vi "Stepper Motor Control.vi"() -> ()   [LabVIEW 2015]
uses:
  <vilib>/MakerHub/LINX/Public/Peripherals/Digital/Digital Write N Chans.vi
  <vilib>/MakerHub/LINX/Private/Local IO/LinxDigitalWrite.vi
  <vilib>/MakerHub/LINX/Public/Utilities/Check Channel.vi
  <vilib>/MakerHub/LINX/Public/Utilities/Open Serial.vi
  <vilib>/MakerHub/LINX/Private/Utilties/Generate Error.vi
  <vilib>/MakerHub/LINX/LMH-LINX.lvlib
panel:
  in  "States":bool[](array[boolean])
  in  "Serial Port":refnum<visa-resource-name>="COM12"
  in  "Stop":bool
  in  "Speed":dbl(slide)=100.0 scale=0.0..200.0
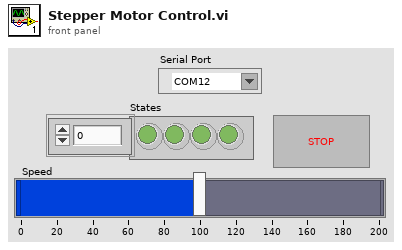
[diagram p1: front panel]
types:
  T1 = typedef "LMH-LINX.lvlib/LINX Ref.ctl" = cluster{"IO":T2, "Interface":T3, "LINX Device Config":T4}
  T2 = typedef "LMH-LINX.lvlib/Platform.ctl" = enum16{"Remote", "Local"}
  T3 = typedef "LMH-LINX.lvlib/Interface.ctl" = enum16{"Serial", "TCP"}
  T4 = typedef "LMH-LINX.lvlib/Device.lvlib/LINX Device Config.ctl" = cluster{"Interface":T3, "COM Port":refnum<visa-resource-name>, "TCP Configuration":T5, "Device Family":u8, "Device ID":u8, "Device Name":string, "TCP Ref":refnum<k5>, "Channels":T6}
  T5 = typedef "LMH-LINX.lvlib/Device.lvlib/TCP Config.ctl" = cluster{"IP Address":string, "Port":u16}
  T6 = typedef "LMH-LINX.lvlib/Channels.ctl" = cluster{"DI":u8[], "DO":u8[], "AI":u8[], "AO":u8[], "PWM":u8[], "QE":u8[], "UART":u8[], "I2C 2":u8[], "SPI":u8[], "CAN":u8[], "Servo":u8[], "AI Ref (V)":dbl, "AI Resolution (Bits)":u8, "AO Ref (V)":dbl, "AO Resolution (Bits)":u8}
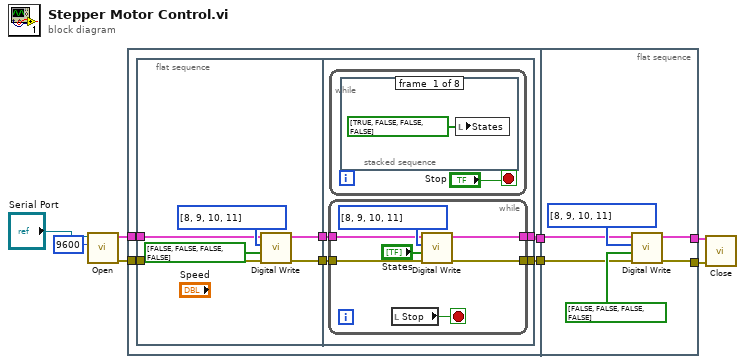
[diagram p0: block diagram]
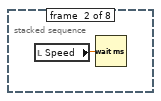
[diagram p2: hidden frame]
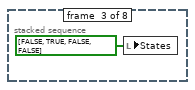
[diagram p3: hidden frame]
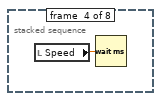
[diagram p4: hidden frame]
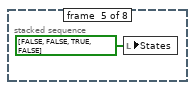
[diagram p5: hidden frame]
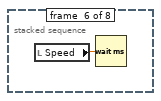
[diagram p6: hidden frame]
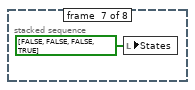
[diagram p7: hidden frame]
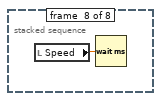
[diagram p8: hidden frame]
diagram:
  n1 = call-poly <vilib>:"Open.vi"("Baud Rate Override"=u32 9600, "Serial Port"="Serial Port") -> ("Error Out"=w7:errorcluster, "LINX Resource"=w8:T1)  [unwired: 7 in, 1 out]
  n2 = flat-sequence {
    tunnel: w8 -> [w14]
    tunnel: w7 -> [w13]
    tunnel: [w10] -> w2
    tunnel: [w9] -> w1
    tunnel: [w44] -> w4
    tunnel: [w43] -> w3
    tunnel: w2 -> [w42]
    tunnel: w1 -> [w41]
    frame #0 {
      n3 = flat-sequence {
        tunnel: w14 -> [w19]
        tunnel: w13 -> [w18]
        tunnel: [w16] -> w12
        tunnel: [w15] -> w11
        tunnel: w12 -> [w24]
        tunnel: w11 -> [w23]
        tunnel: [w22] -> w10
        tunnel: [w21] -> w9
        frame #0 {
          n4 = call-poly <vilib>:"Digital Write.vi"("Error In"=w18, "Values"=bool[] [FALSE, FALSE, FALSE, FALSE] ("State 1"), "DO Channels"=u8[] [8, 9, 10, 11], "LINX Resource"=w19) -> ("Error Out"=w15:errorcluster, "LINX Resource"=w16:T1)  [unwired: 6 in]
        }
        frame #1 {
          n5 = while {
            tunnel: w24 -> [w38]
            tunnel: w23 -> [w37]
            tunnel: [w36] -> w22
            tunnel: [w35] -> w21
            stop <- w34 stop-if-true
            n6 = local read "Stop"() -> (w34:bool)
            n7 = call-poly <vilib>:"Digital Write.vi"("Error In"=w37, "Values"="States", "DO Channels"=u8[] [8, 9, 10, 11], "LINX Resource"=w38) -> ("Error Out"=w35:errorcluster, "LINX Resource"=w36:T1)  [unwired: 6 in]
          }
          n8 = while {
            stop <- "Stop" stop-if-true
            n9 = stacked-sequence {
              frame #0 {
                n10 = local write "States"(bool[] [TRUE, FALSE, FALSE, FALSE] ("Values")) -> ()
              }
              frame #1 {
                n11 = local read "Speed"() -> (w27:dbl)
                n12 = Wait (ms)(milliseconds to wait=w27) -> ()  [unwired: 1 out]
              }
              frame #2 {
                n13 = local write "States"(bool[] [FALSE, TRUE, FALSE, FALSE] ("Values")) -> ()
              }
              frame #3 {
                n14 = local read "Speed"() -> (w29:dbl)
                n15 = Wait (ms)(milliseconds to wait=w29) -> ()  [unwired: 1 out]
              }
              frame #4 {
                n16 = local write "States"(bool[] [FALSE, FALSE, TRUE, FALSE] ("Values")) -> ()
              }
              frame #5 {
                n17 = local read "Speed"() -> (w31:dbl)
                n18 = Wait (ms)(milliseconds to wait=w31) -> ()  [unwired: 1 out]
              }
              frame #6 {
                n19 = local write "States"(bool[] [FALSE, FALSE, FALSE, TRUE] ("Values")) -> ()
              }
              frame #7 {
                n20 = local read "Speed"() -> (w33:dbl)
                n21 = Wait (ms)(milliseconds to wait=w33) -> ()  [unwired: 1 out]
              }
            }
          }
        }
      }
    }
    frame #1 {
      n22 = call-poly <vilib>:"Digital Write.vi"("Error In"=w41, "Values"=bool[] [FALSE, FALSE, FALSE, FALSE] ("States 2"), "DO Channels"=u8[] [8, 9, 10, 11], "LINX Resource"=w42) -> ("Error Out"=w43:errorcluster, "LINX Resource"=w44:T1)  [unwired: 6 in]
    }
  }
  n23 = call <vilib>:"Close.vi"("Error In"=w3, "LINX Resource"=w4) -> ()  [unwired: 9 in, 1 out]
